vi "Configure Trigger.vi"(0 "VISA resource name":refnum<visa-resource-name>, 1 "Trigger Count (1)":i32=1, 2 "Enable Setting-time Delay (F: Disable)":bool, 5 "Trigger Level (0 dBm)":dbl, 7 "Trigger Slope (0: Positive)":u16(ring) items=["Positive", "Negative"], 9 "Trigger Source (3: Immediate)":i32(ring)=3 items=["Bus", "External", "Hold", "Immediate", "Internal A"], 11 "error in (no error)":errorcluster, 12 "Trigger Hysteresis (0 dB)":dbl) -> (4 "VISA resource name out":refnum<visa-resource-name>, 15 "error out":errorcluster)   [LabVIEW 2018, in "Agilent U2000 Series.lvlib"]
doc: "Controls the behavior of the trigger system, including Trigger Source, Trigger Slope,Trigger Level, Trigger Delay, Trigger Count and Hysteresis."
uses:
  Agilent U2000 Series.lvlib
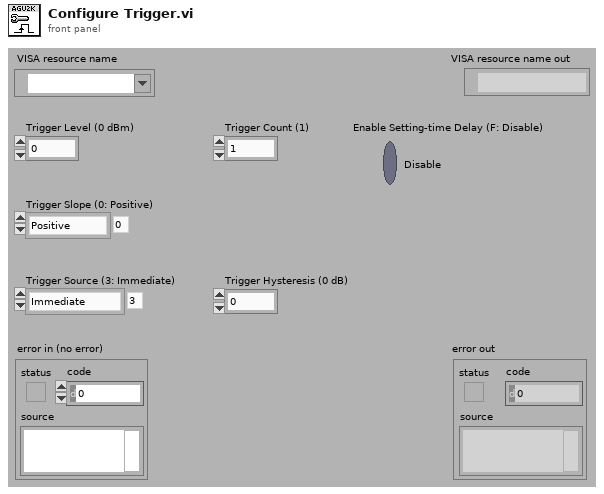
[diagram p1: front panel]
types:
  T1 = typedef "Agilent U2000 Series.lvlib/Extended User Data.ctl" = cluster{"U2000 Series Mode":u16, "Trigger Source Int/Ext":bool}
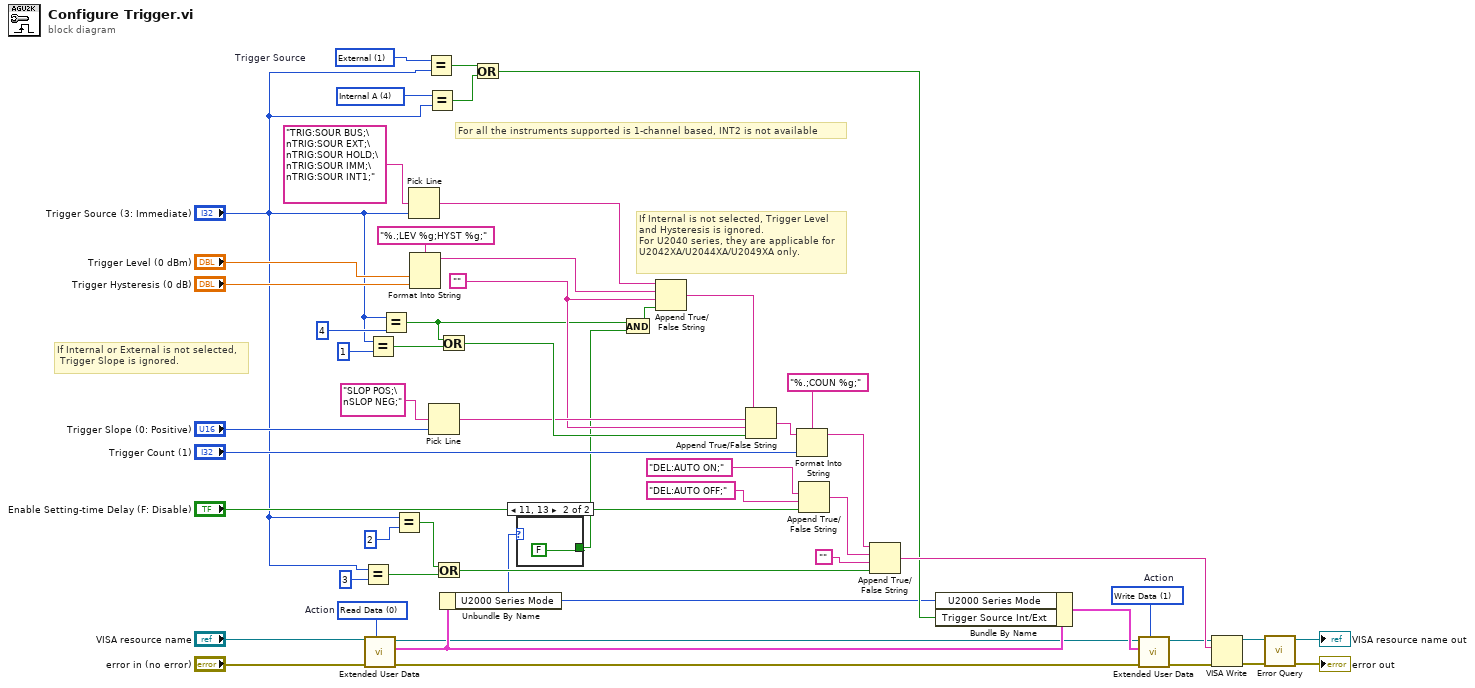
[diagram p0: block diagram]
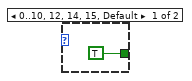
[diagram p2: hidden frame]
diagram:
  w16 = 0 items=["Read Data", "Write Data", "Clear Data", "Clear ALL Data"]  # Action
  w17 = 1 items=["Read Data", "Write Data", "Clear Data", "Clear ALL Data"]  # Action
  w18 = 4 items=["Bus", "External", "Hold", "Immediate", "Internal A"] ("Trigger Source (3: Immediate)")
  w19 = 1 items=["Bus", "External", "Hold", "Immediate", "Internal A"]  # Trigger Source
  w38 = ""
  # "If Internal or External is not selected,\n Trigger Slope is ignored."
  # "If Internal is not selected, Trigger Level and Hysteresis is ignored.\nFor U2040 series, they are applicable for U2042XA/U2044XA/U2049XA only."
  # "For all the instruments supported is 1-channel based, INT2 is not available"
  n1 = Equal?(x="Trigger Source (3: Immediate)", y=3) -> (x = y?=w34:bool)
  n2 = call "Extended User Data.vi"("Action (1: Write Data)"=w16, "error in (no error)"="error in (no error)", "VISA resource name"="VISA resource name") -> ("error out"=w9:errorcluster, "User Data Out"=w12:T1, "VISA resource name out"=w10:refnum<visa-resource-name>)  [unwired: 1 in, 5 out]
  n3 = Equal?(x="Trigger Source (3: Immediate)", y=1) -> (x = y?=w5:bool)
  n4 = Equal?(x="Trigger Source (3: Immediate)", y=4) -> (x = y?=w4:bool)
  n5 = Equal?(x="Trigger Source (3: Immediate)", y=2) -> (x = y?=w35:bool)
  n6 = Pick Line(multi-line string="TRIG:SOUR BUS;\nTRIG:SOUR EXT;\nTRIG:SOUR HOLD;\nTRIG:SOUR IMM;\nTRIG:SOUR INT1;", line index="Trigger Source (3: Immediate)") -> (output string=w30:string)  [unwired: 1 out]
  n7 = Format Into String(format string="%.;LEV %g;HYST %g;", "Trigger Level (0 dBm)", "Trigger Hysteresis (0 dB)") -> (resulting string=w42:string)  [unwired: 2 in, 1 out]
  n8 = Equal?(x=w19, y="Trigger Source (3: Immediate)") -> (x = y?=w21:bool)
  n9 = Equal?(x=w18, y="Trigger Source (3: Immediate)") -> (x = y?=w20:bool)
  n10 = Pick Line(multi-line string="SLOP POS;\nSLOP NEG;", line index="Trigger Slope (0: Positive)") -> (output string=w40:string)  [unwired: 1 out]
  n11 = Or(x=w35, y=w34) -> (x .or. y?=w33:bool)
  n12 = Or(x=w4, y=w5) -> (x .or. y?=w43:bool)
  n13 = Unbundle By Name(w12) -> ("U2000 Series Mode"=w1:u16)
  n14 = Or(x=w21, y=w20) -> (x .or. y?=w15:bool)
  n15 = case shown="11, 13" w1 {
    tunnel: [TRUE FALSE] -> w2
    frame 0..10, 12, 14, 15, Default {
    }
    frame 11, 13 {
    }
  }
  n16 = And(x=w4, y=w2) -> (x .and. y?=w3:bool)
  n17 = Append True/False String(1:w3, 2:w38, 3:w42, 4:w30) -> (0:w41:string)
  n18 = Append True/False String(1:w43, 2:w38, 3:w40, 4:w41) -> (0:w27:string)
  n19 = Format Into String(format string="%.;COUN %g;", initial string=w27, "Trigger Count (1)") -> (resulting string=w26:string)  [unwired: 1 in, 1 out]
  n20 = Append True/False String(1:"Enable Setting-time Delay (F: Disable)", 2:"DEL:AUTO OFF;", 3:"DEL:AUTO ON;") -> (0:w28:string)  [unwired: 1 out]
  n21 = Append True/False String(1:w33, 2:"", 3:w28, 4:w26) -> (0:w29:string)
  n22 = Bundle By Name(cluster=w12, "U2000 Series Mode"=w1, "Trigger Source Int/Ext"=w15) -> (w11:T1)
  n23 = call "Extended User Data.vi"("Action (1: Write Data)"=w17, "error in (no error)"=w9, "User Data In"=w11, "VISA resource name"=w10) -> ("error out"=w7:errorcluster, "VISA resource name out"=w8:refnum<visa-resource-name>)  [unwired: 6 out]
  n24 = VISA Write(VISA resource name=w8, write buffer=w29, error in (no error)=w7) -> (VISA resource name out=w24:refnum<visa-resource-name>, error out=w25:errorcluster)  [unwired: 1 out]
  n25 = call "Error Query.vi"("error in (no error)"=w25, "VISA resource name"=w24) -> ("error out"=→"error out":errorcluster, "VISA resource name out"=→"VISA resource name out":refnum<visa-resource-name>)  [unwired: 8 out]
